vi "GetCtlRef.vi"(8 "Error in":errorcluster, 10 "CtlName In":string, 11 "CtlLookup In":T1) -> (0 "error out":errorcluster, 1 "CtlRef":refnum<vi>, 2 "CtlName Out":string, 3 "CtlLookup Out":T1)   [LabVIEW 2020, in "CtlReferences.lvlib" / "CtlReferences.lvclass"]
uses:
  CtlReferences.lvclass
  TypeDefs/CtlLookup.ctl
  <vilib>/Utility/error.llb/Error Cluster From Error Code.vi
  CtlReferences.lvclass/CtlReferences.ctl
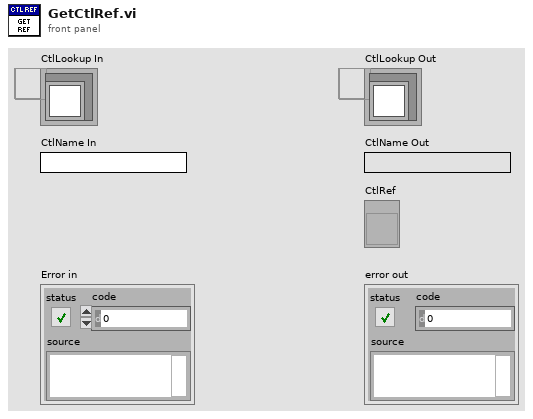
[diagram p1: front panel]
types:
  T1 = typedef "CtlReferences.lvlib/CtlReferences.lvclass/CtlLookup.ctl" = refnum<data-value>
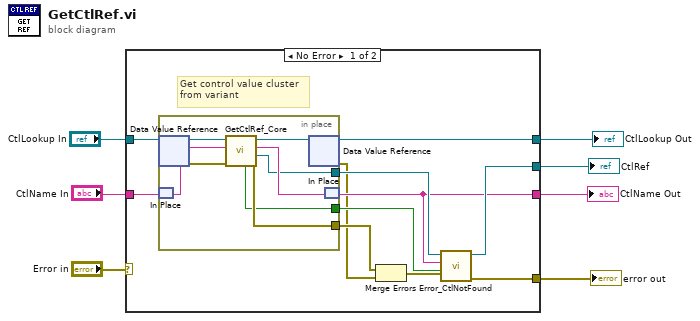
[diagram p0: block diagram]
diagram:
  n1 = case shown="No Error" "Error in" {
    selector: "Error in" -> [_ w29]
    tunnel: [w18 w28] -> w7
    tunnel: "CtlName In" -> [w17 w27]
    tunnel: "CtlLookup In" -> [w16 w28]
    tunnel: [w14 w29] -> w4
    tunnel: [w12 _] -> w3
    tunnel: [w11 w27] -> w2
    frame No Error {
      # "Get control value cluster\nfrom variant"
      n2 = in-place {
        in-place-border: [w20] -> w13
        in-place-border: [w25] -> w9
        in-place-border: [w19] -> w10
        n3 = in-place-dvr #1(w16) -> (w24:refnum<class "CtlReferences.lvclass">, w26:errorcluster)
        n4 = in-place-match #2(w17) -> (w22:string)
        n5 = call-dynamic "GetCtlRef_Core.vi"("error in (no error)"=w26, "CtlName In"=w22, "CtlReferences in"=w24) -> ("error out"=w25:errorcluster, "Ctl Refnum"=w20:refnum<vi>, "CtlName out"=w21:string, "CtlReferences out"=w23:refnum<class "CtlReferences.lvclass">, "Found"=w19:bool)  [unwired: 4 in]
        n6 = in-place-dvr #1(w23) -> (w18:T1, w8:errorcluster)
        n7 = in-place-match #2(w21) -> (w11:string)
      }
      n8 = Merge Errors(w9, w8) -> (w15:errorcluster)
      n9 = call "Error_CtlNotFound.vi"("error in (no error)"=w15, "Control Found?"=w10, "CtlName"=w11, "Control in"=w13) -> ("error out"=w14:errorcluster, "Control out"=w12:refnum<vi>)  [unwired: 6 in]
    }
    frame Error {
    }
  }
  "error out" <- w4
  "CtlName Out" <- w2
  "CtlLookup Out" <- w7
  "CtlRef" <- w3
